vi "Read Config.vi"(8 "error in (no error)":errorcluster, 11 "SequencerInfo in":refnum<class "SequencerInfo.lvclass">) -> (0 "error out":errorcluster, 2 "Sequencer.lvlib:SequencerConfig.lvclass":refnum<class "SequencerConfig.lvclass">, 3 "SequencerInfo out":refnum<class "SequencerInfo.lvclass">)   [LabVIEW 2015, in "Sequencer.lvlib" / "SequencerInfo.lvclass"]
uses:
  SequencerInfo.lvclass
  SequencerConfig.lvclass
  SequencerInfo.lvclass/SequencerInfo.ctl
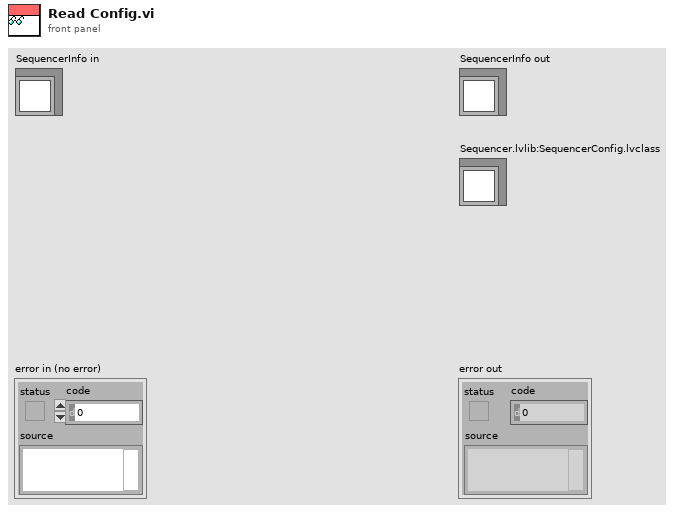
[diagram p1: front panel]
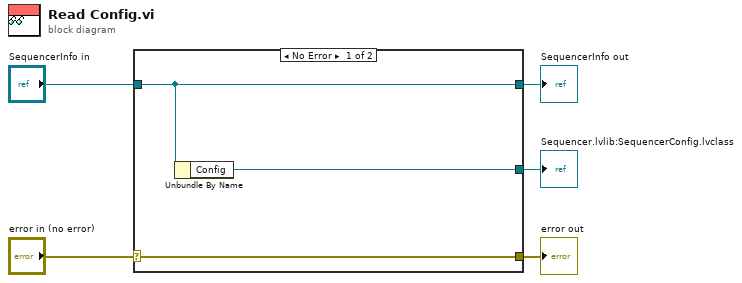
[diagram p0: block diagram]
diagram:
  n1 = case shown="No Error" "error in (no error)" {
    selector: "error in (no error)" -> [w8 w9]
    tunnel: [w8 w9] -> w4
    tunnel: [w7 w10] -> w2
    tunnel: "SequencerInfo in" -> [w7 w10]
    tunnel: [w6 _] -> w1
    frame No Error {
      n2 = Unbundle By Name(w7) -> ("Config"=w6:refnum<class "SequencerConfig.lvclass">)
    }
    frame Error {
    }
  }
  "error out" <- w4
  "SequencerInfo out" <- w2
  "Sequencer.lvlib:SequencerConfig.lvclass" <- w1
